vi "SMU_Single Channel Meas.vi"(7 "Meas_A_Level":dbl, 8 "error in (no error)":errorcluster, 9 "Published Data Id":string, 10 "Pins":string[](array[string]), 11 "Semiconductor Module Context":T1) -> (0 "error Out":errorcluster, 2 "R Array":dbl[](array[numeric]), 3 "Semiconductor Module Context Out":T1)   [LabVIEW 2013]
uses:
  <vilib>/NI_TestStand_SemiconductorModule/NI_TestStand_Semiconductor_Module.lvlibp/PinMap/General/SemiconductorModuleContext.ctl
  <vilib>/NI_TestStand_SemiconductorModule/NI_TestStand_Semiconductor_Module.lvlibp/PinMap/DC Power/PinsToNIDCPowerSessions.vi
  <vilib>/NI_TestStand_SemiconductorModule/NI_TestStand_Semiconductor_Module.lvlibp/PinMap/General/Publish/PublishDataDoubleFunctionalTest.vi
  <vilib>/NI_TestStand_SemiconductorModule/NI_TestStand_Semiconductor_Module.lvlibp
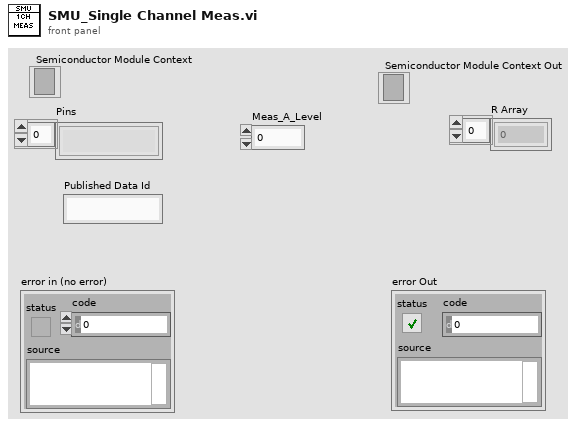
[diagram p1: front panel]
types:
  T1 = typedef "NI_TestStand_Semiconductor_Module.lvlibp/SemiconductorModuleContext.ctl" = refnum<k7>
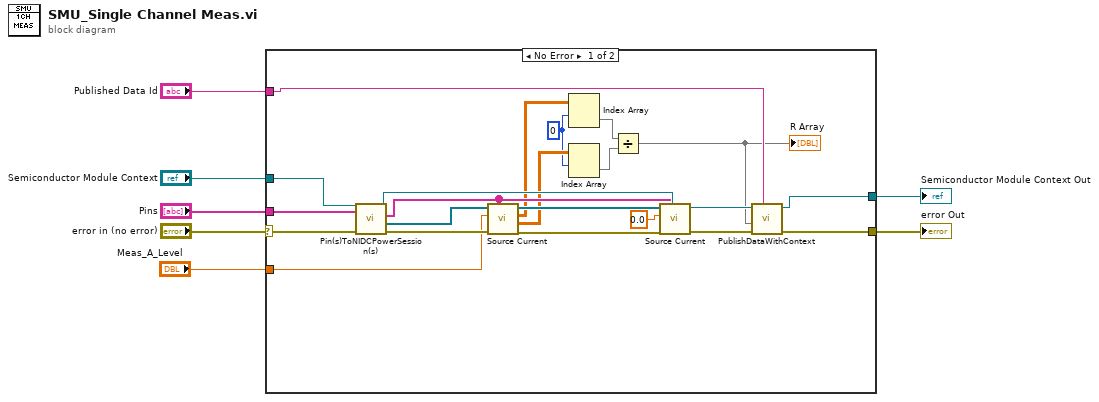
[diagram p0: block diagram]
diagram:
  n1 = case shown="No Error" "error in (no error)" {
    selector: "error in (no error)" -> [w27 w30]
    tunnel: "Semiconductor Module Context" -> [w24 w29]
    tunnel: "Pins" -> [w25 _]
    tunnel: [w23 w30] -> w4
    tunnel: "Published Data Id" -> [w28 _]
    tunnel: [w26 w29] -> w2
    tunnel: "Meas_A_Level" -> [w8 _]
    frame No Error {
      w12 = 0 ("index (row)")
      n2 = call-poly <vilib>:"Pin(s)ToNIDCPowerSession(s).vi"("error in (no error)"=w27, "Pins"=w25, "Semiconductor Module Context"=w24) -> ("error out"=w19:errorcluster, "Instrument Sessions"=w20:refnum<k15>[], "Channel Lists"=w17:string[], "Semiconductor Module Context Out"=w18:T1)  [unwired: 4 in, 1 out]
      n3 = call "Source Current.vi"("Channel Lists"=w17, "error in (no error)"=w19, "current level"=w8, "Instrument Sessions In"=w20) -> ("error out"=w16:errorcluster, "current measurements"=w13:dbl[][], "voltage measurements"=w14:dbl[][], "Instrument Sessions Out"=w15:refnum<k15>[])  [unwired: 4 in]
      n4 = Index Array(array=w14, index (row)=w12) -> (element=w11:dbl[])  [unwired: 1 in]
      n5 = Index Array(array=w13, index (row)=w12) -> (element=w10:dbl[])  [unwired: 1 in]
      n6 = Divide(x=w11, y=w10) -> (x/y=w9:dbl[])
      "R Array" <- w9
      n7 = call "Source Current.vi"("Channel Lists"=w17, "error in (no error)"=w16, "current level"=0.0, "Instrument Sessions In"=w15) -> ("error out"=w21:errorcluster)  [unwired: 4 in, 3 out]
      n8 = call-poly <vilib>:"PublishDataWithContext.vi"("Published Data Id"=w28, "error in (no error)"=w21, "Data In"=w9, "Semiconductor Module Context"=w18) -> ("error out"=w23:errorcluster, "Semiconductor Module Context Out"=w26:T1)  [unwired: 6 in]
    }
    frame Error {
    }
  }
  "error Out" <- w4
  "Semiconductor Module Context Out" <- w2
